vi "InitConfigLCR.vi"(0 "VISA resource name LCR":refnum<visa-resource-name>, 1 "Short (F:OFF)":bool, 2 "Open (F:OFF)":bool, 5 "Imp Type (0: CPD)":u32(ring) items=["CPD", "CPQ", "CPG", "CPRP", "CSD", "CSQ", "CSRS", "LPQ", "LPD", "LPG", "LPRP", "LSD", "LSQ", "LSRS", "RX", "ZTD", "ZTR", "GB", "YTD", "YTR"], 7 "Freq Value (Hz)(1.0 kHz)":dbl=1000.0 min=20.0 max=30000000.0 step=10.0 format="%.4e", 9 "Voltage Level (V)(1.0V)":dbl=1.0 min=0.0 max=20.0 step=0.1 format="%.4f", 11 "error in (no error)":errorcluster) -> (4 "VISA resource name out":refnum<visa-resource-name>, 15 "error out":errorcluster)   [LabVIEW 2016]
uses:
  <instrlib>/Agilent 428X Series/Agilent 428X Series.lvlib
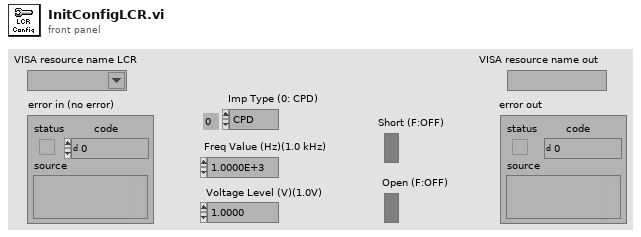
[diagram p1: front panel]
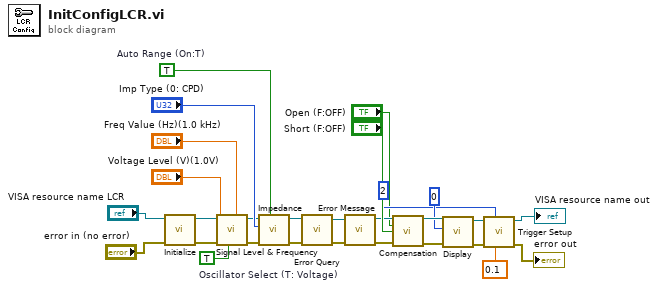
[diagram p0: block diagram]
diagram:
  w11 = TRUE  # Oscillator Select (T: Voltage)
  w7 = TRUE  # Auto Range (On:T)
  n1 = call <instrlib>:"Initialize.vi"("error in (no error)"="error in (no error)", "VISA resource name"="VISA resource name LCR") -> ("error out"=w19:errorcluster, "VISA resource name out"=w18:refnum<visa-resource-name>)  [unwired: 8 in]
  n2 = call <instrlib>:"Signal Level & Frequency.vi"("Frequency Value (Hz) (100KHz)"="Freq Value (Hz)(1.0 kHz)", "Oscillator Select (T: Voltage)"=w11, "error in (no error)"=w19, "Voltage Level (V) (5mV)"="Voltage Level (V)(1.0V)", "VISA resource name"=w18) -> ("error out"=w6:errorcluster, "VISA resource name out"=w5:refnum<visa-resource-name>)  [unwired: 5 in]
  n3 = call <instrlib>:"Impedance.vi"("Auto Range (F: Off)"=w7, "error in (no error)"=w6, "Imp Type (0: CPD)"="Imp Type (0: CPD)", "VISA resource name"=w5) -> ("error out"=w12:errorcluster, "VISA resource name out"=w13:refnum<visa-resource-name>)  [unwired: 6 in]
  n4 = call <instrlib>:"Error Query.vi"("error in (no error)"=w12, "VISA resource name"=w13) -> ("error out"=w20:errorcluster, "VISA resource name out"=w14:refnum<visa-resource-name>)  [unwired: 6 in, 2 out]
  n5 = call <instrlib>:"Error Message.vi"("error in (no error)"=w20, "VISA resource name"=w14) -> ("error out"=w15:errorcluster, "VISA resource name out"=w16:refnum<visa-resource-name>)  [unwired: 5 in, 3 out]
  n6 = call <instrlib>:"Compensation.VI"("VISA resource name"=w16, "OPEN (F:OFF)"="Open (F:OFF)", "SHORT (F:OFF)"="Short (F:OFF)", "error in (no error)"=w15) -> ("VISA resource name out"=w27:refnum<visa-resource-name>, "error out"=w26:errorcluster)  [unwired: 10 in]
  n7 = call <instrlib>:"Display.vi"("error in (no error)"=w26, "Display Page (0: Measurement)"=u32 0 ("Display Page (Measurment:0)"), "VISA resource name"=w27) -> ("error out"=w24:errorcluster, "VISA resource name out"=w25:refnum<visa-resource-name>)  [unwired: 7 in]
  n8 = call <instrlib>:"Trigger Setup.vi"("Delay Value (s) (0.0)"=0.1, "Trigger Source (0: Internal)"=u32 2 ("bus triggering"), "error in (no error)"=w24, "VISA resource name"=w25) -> ("error out"=→"error out":errorcluster, "VISA resource name out"=→"VISA resource name out":refnum<visa-resource-name>)  [unwired: 6 in]
